vi "Get Temporary Config File Path.vi"(8 "error in (no error)":errorcluster, 11 "Base Test in":refnum<class "Process Test.lvclass">) -> (0 "error out":errorcluster, 2 "Temporary Config File Path":path, 3 "Base Test out":refnum<class "Process Test.lvclass">)   [LabVIEW 2020, in "Process Test.lvclass"]
uses:
  Process Test.lvclass
  Process Test.lvclass/Process Test.ctl
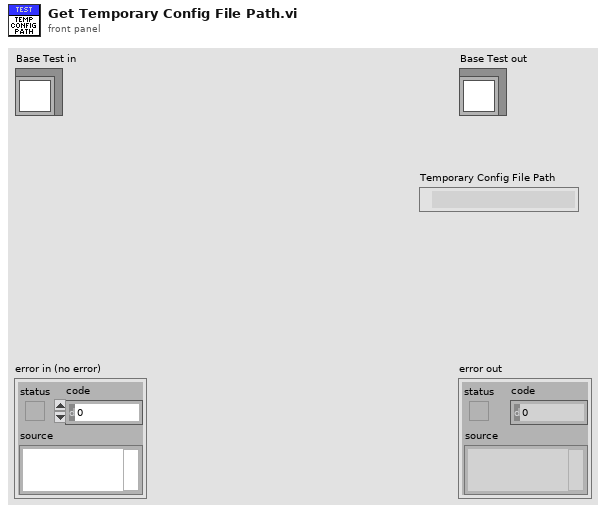
[diagram p1: front panel]
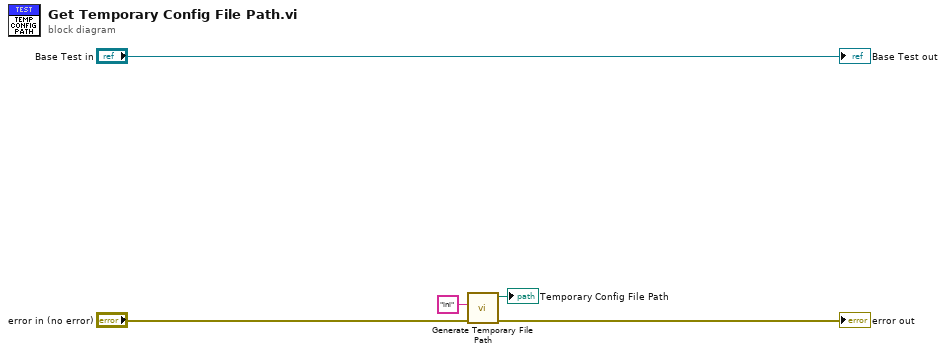
[diagram p0: block diagram]
diagram:
  n1 = call <vilib>:"Generate Temporary File Path.vi"("error in (no error)"="error in (no error)", "Temporary File Extension (tmp)"="ini") -> ("error out"=→"error out":errorcluster, "Unique Temporary File Path"=→"Temporary Config File Path":path)  [unwired: 8 in]
  "Base Test out" <- "Base Test in"
